vi "HFRR ADV v015 new software.vi"() -> ()   [LabVIEW 2025] (continued)
              n2034 = String Subset(string=w2234, offset (0)=35, length (rest)=9 ("length (rest)")) -> (substring=w2257:string)
              n2035 = String Subset(string=w2234, offset (0)=55, length (rest)=9 ("length (rest)")) -> (substring=w2242:string)
              n2036 = String Subset(string=w2234, offset (0)=25) -> (substring=w2238:string)  [unwired: 1 in]
              n2037 = String Subset(string=w2234, offset (0)=15, length (rest)=9 ("length (rest)")) -> (substring=w2263:string)
              n2038 = String Subset(string=w2234, offset (0)=0, length (rest)=14 ("length (rest)")) -> (substring=w2260:string)
              n2039 = String Subset(string=w2234, offset (0)=45, length (rest)=9 ("length (rest)")) -> (substring=w2247:string)
              n2040 = String Subset(string=w2234, offset (0)=65, length (rest)=9 ("length (rest)")) -> (substring=w2253:string)
              n2041 = Fract/Exp String To Number(string=w2236) -> (number=w2233:dbl)  [unwired: 3 in, 1 out]
              n2042 = Fract/Exp String To Number(string=w2257) -> (number=w2255:dbl)  [unwired: 3 in, 1 out]
              n2043 = Fract/Exp String To Number(string=w2242) -> (number=w2240:dbl)  [unwired: 3 in, 1 out]
              n2044 = Fract/Exp String To Number(string=w2238) -> (number=w2237:dbl)  [unwired: 3 in, 1 out]
              n2045 = Fract/Exp String To Number(string=w2263) -> (number=w2254:dbl)  [unwired: 3 in, 1 out]
              n2046 = Fract/Exp String To Number(string=w2260) -> (number=w2256:dbl)  [unwired: 3 in, 1 out]
              n2047 = Fract/Exp String To Number(string=w2247) -> (number=w2244:dbl)  [unwired: 3 in, 1 out]
              n2048 = Fract/Exp String To Number(string=w2253) -> (number=w2250:dbl)  [unwired: 3 in, 1 out]
              n2049 = Add(x=w2250, y=0.0) -> (x+y=w2248:dbl)
            }
            n2050 = String To Path(string=w2093) -> (path=w2191:path)
            n2051 = String To Path(string=w2091) -> (path=w2185:path)
            n2052 = local read "Numeric 11"() -> (w2175:i32)
            n2053 = local read "Numeric 13"() -> (w2177:i32)
            n2054 = Open/Create/Replace File "Open File"(file path (use dialog)=w2191) -> (refnum out=w2189:refnum<file>, error out=w2188:errorcluster)  [unwired: 5 in, 1 out]
            n2055 = Open/Create/Replace File "Open File"(file path (use dialog)=w2185) -> (refnum out=w2184:refnum<file>, error out=w2183:errorcluster)  [unwired: 5 in, 1 out]
            n2056 = for {
              N: w2175 -> [_]
              tunnel: w2189 -> [w2304]
              tunnel: w2188 -> [w2303]
              tunnel: [w2293] -> w2155 mode=indexing
              tunnel: [w2291] -> w2153 mode=indexing
              tunnel: [w2292] -> w2148 mode=indexing
              tunnel: w2174 -> [_]
              tunnel: [w2285] -> w2150 mode=indexing
              tunnel: [w2281] -> w2126 mode=indexing
              tunnel: [w2277] -> w2101 mode=indexing
              tunnel: [w2273] -> w2082 mode=indexing
              tunnel: [w2268] -> w2040 mode=indexing
              (unwired) TRUE ("line mode (F)")
              n2057 = Read from Text File "Read File"(file (use dialog)=w2304, error in=w2303) -> (text=w2269:string)  [unwired: 2 in, 3 out]
              n2058 = local write "String 7"(w2269) -> ()
              n2059 = String Subset(string=w2269, offset (0)=85, length (rest)=9 ("length (rest)")) -> (substring=w2272:string)
              n2060 = String Subset(string=w2269, offset (0)=35, length (rest)=9 ("length (rest)")) -> (substring=w2294:string)
              n2061 = String Subset(string=w2269, offset (0)=55, length (rest)=9 ("length (rest)")) -> (substring=w2280:string)
              n2062 = String Subset(string=w2269, offset (0)=25, length (rest)=9 ("length (rest)")) -> (substring=w2274:string)
              n2063 = String Subset(string=w2269, offset (0)=45, length (rest)=9 ("length (rest)")) -> (substring=w2282:string)
              n2064 = String Subset(string=w2269, offset (0)=0, length (rest)=14 ("length (rest)")) -> (substring=w2297:string)
              n2065 = String Subset(string=w2269, offset (0)=15, length (rest)=9 ("length (rest)")) -> (substring=w2300:string)
              n2066 = String Subset(string=w2269, offset (0)=65, length (rest)=9 ("length (rest)")) -> (substring=w2286:string)
              n2067 = Fract/Exp String To Number(string=w2272) -> (number=w2268:dbl)  [unwired: 3 in, 1 out]
              n2068 = Fract/Exp String To Number(string=w2294) -> (number=w2292:dbl)  [unwired: 3 in, 1 out]
              n2069 = Fract/Exp String To Number(string=w2280) -> (number=w2277:dbl)  [unwired: 3 in, 1 out]
              n2070 = Fract/Exp String To Number(string=w2274) -> (number=w2273:dbl)  [unwired: 3 in, 1 out]
              n2071 = Fract/Exp String To Number(string=w2282) -> (number=w2281:dbl)  [unwired: 3 in, 1 out]
              n2072 = Fract/Exp String To Number(string=w2297) -> (number=w2293:dbl)  [unwired: 3 in, 1 out]
              n2073 = Fract/Exp String To Number(string=w2300) -> (number=w2291:dbl)  [unwired: 3 in, 1 out]
              n2074 = Fract/Exp String To Number(string=w2286) -> (number=w2289:dbl)  [unwired: 3 in, 1 out]
              n2075 = Add(x=w2289, y=0.0) -> (x+y=w2285:dbl)
            }
            n2076 = for {
              N: w2177 -> [_]
              tunnel: w2184 -> [w2232]
              tunnel: w2183 -> [w2231]
              tunnel: [w2221] -> w2137 mode=indexing
              tunnel: [w2220] -> w2130 mode=indexing
              tunnel: w2174 -> [_]
              tunnel: [w2209] -> w2135 mode=indexing
              tunnel: [w2214] -> w2132 mode=indexing
              tunnel: [w2210] -> w2122 mode=indexing
              tunnel: [w2205] -> w2097 mode=indexing
              tunnel: [w2201] -> w2078 mode=indexing
              tunnel: [w2196] -> w2038 mode=indexing
              (unwired) 1.0 ("x")
              (unwired) TRUE ("line mode (F)")
              n2077 = Read from Text File "Read File"(file (use dialog)=w2232, error in=w2231) -> (text=w2197:string)  [unwired: 2 in, 3 out]
              n2078 = local write "String 12"(w2197) -> ()
              n2079 = String Subset(string=w2197, offset (0)=85, length (rest)=9 ("length (rest)")) -> (substring=w2199:string)
              n2080 = String Subset(string=w2197, offset (0)=35, length (rest)=9 ("length (rest)")) -> (substring=w2222:string)
              n2081 = String Subset(string=w2197, offset (0)=55, length (rest)=9 ("length (rest)")) -> (substring=w2207:string)
              n2082 = String Subset(string=w2197, offset (0)=25, length (rest)=9 ("length (rest)")) -> (substring=w2203:string)
              n2083 = String Subset(string=w2197, offset (0)=45, length (rest)=9 ("length (rest)")) -> (substring=w2212:string)
              n2084 = String Subset(string=w2197, offset (0)=15, length (rest)=9 ("length (rest)")) -> (substring=w2228:string)
              n2085 = String Subset(string=w2197, offset (0)=0, length (rest)=14 ("length (rest)")) -> (substring=w2225:string)
              n2086 = String Subset(string=w2197, offset (0)=65, length (rest)=9 ("length (rest)")) -> (substring=w2215:string)
              n2087 = Fract/Exp String To Number(string=w2199) -> (number=w2196:dbl)  [unwired: 3 in, 1 out]
              n2088 = Fract/Exp String To Number(string=w2222) -> (number=w2220:dbl)  [unwired: 3 in, 1 out]
              n2089 = Fract/Exp String To Number(string=w2207) -> (number=w2205:dbl)  [unwired: 3 in, 1 out]
              n2090 = Fract/Exp String To Number(string=w2203) -> (number=w2201:dbl)  [unwired: 3 in, 1 out]
              n2091 = Fract/Exp String To Number(string=w2212) -> (number=w2210:dbl)  [unwired: 3 in, 1 out]
              n2092 = Fract/Exp String To Number(string=w2228) -> (number=w2209:dbl)  [unwired: 3 in, 1 out]
              n2093 = Fract/Exp String To Number(string=w2225) -> (number=w2221:dbl)  [unwired: 3 in, 1 out]
              n2094 = Fract/Exp String To Number(string=w2215) -> (number=w2218:dbl)  [unwired: 3 in, 1 out]
              n2095 = Add(x=w2218, y=0.0) -> (x+y=w2214:dbl)
            }
            n2096 = Delete From Array(array=w2080, index=0) -> (array with subset deleted=w2053:dbl[])  [unwired: 1 in, 1 out]
            n2097 = Delete From Array(array=w2143, index=0) -> (array with subset deleted=w2116:dbl[])  [unwired: 1 in, 1 out]
            n2098 = Delete From Array(array=w2123, index=0) -> (array with subset deleted=w2111:dbl[])  [unwired: 1 in, 1 out]
            n2099 = Delete From Array(array=w2141, index=0) -> (array with subset deleted=w2142:dbl[])  [unwired: 1 in, 1 out]
            n2100 = call-poly <vilib>:"Mean.vi"("X"=w2053) -> ("mean"=→"КОФ2 4":dbl)  [unwired: 1 out]
            n2101 = call-poly <vilib>:"Mean.vi"("X"=w2116) -> ("mean"=→"КОФ3":dbl)  [unwired: 1 out]
            n2102 = call-poly <vilib>:"Mean.vi"("X"=w2111) -> ("mean"=→"CP3":dbl)  [unwired: 1 out]
            n2103 = Delete From Array(array=w2105, index=0) -> (array with subset deleted=w2032:dbl[])  [unwired: 1 in, 1 out]
            n2104 = Delete From Array(array=w2044, index=0) -> (array with subset deleted=w2031:dbl[])  [unwired: 1 in, 1 out]
            n2105 = Delete From Array(array=w2084, index=0) -> (array with subset deleted=w2055:dbl[])  [unwired: 1 in, 1 out]
            n2106 = Delete From Array(array=w2162, index=0) -> (array with subset deleted=w2117:dbl[])  [unwired: 1 in, 1 out]
            n2107 = Delete From Array(array=w2128, index=0) -> (array with subset deleted=w2113:dbl[])  [unwired: 1 in, 1 out]
            "array w/ subset deleted" <- w2113
            n2108 = Delete From Array(array=w2159, index=0) -> (array with subset deleted=w2160:dbl[])  [unwired: 1 in, 1 out]
            n2109 = call-poly <vilib>:"Mean.vi"("X"=w2055) -> ("mean"=→"КОФ2 2":dbl)  [unwired: 1 out]
            n2110 = call-poly <vilib>:"Mean.vi"("X"=w2117) -> ("mean"=→"КОФ1":dbl)  [unwired: 1 out]
            n2111 = Bundle "Bundle"(w2032, w2031) -> (w2037:cluster{dbl[], dbl[]})  [unwired: 1 in]
            n2112 = Bundle "Bundle"(w2032, w2160) -> (w2024:cluster{dbl[], dbl[]})  [unwired: 1 in]
            n2113 = Delete From Array(array=w2039, index=0) -> (array with subset deleted=w2027:dbl[])  [unwired: 1 in, 1 out]
            n2114 = Delete From Array(array=w2040, index=0) -> (array with subset deleted=w2029:dbl[])  [unwired: 1 in, 1 out]
            n2115 = Delete From Array(array=w2150, index=0) -> (array with subset deleted=w2151:dbl[])  [unwired: 1 in, 1 out]
            n2116 = Delete From Array(array=w2038, index=0) -> (array with subset deleted=w2025:dbl[])  [unwired: 1 in, 1 out]
            n2117 = Delete From Array(array=w2132, index=0) -> (array with subset deleted=w2133:dbl[])  [unwired: 1 in, 1 out]
            n2118 = Delete From Array(array=w2157, index=0) -> (array with subset deleted=w2063:dbl[])  [unwired: 1 in, 1 out]
            n2119 = Delete From Array(array=w2103, index=0) -> (array with subset deleted=w2059:dbl[])  [unwired: 1 in, 1 out]
            n2120 = Delete From Array(array=w2139, index=0) -> (array with subset deleted=w2061:dbl[])  [unwired: 1 in, 1 out]
            n2121 = Delete From Array(array=w2099, index=0) -> (array with subset deleted=w2057:dbl[])  [unwired: 1 in, 1 out]
            n2122 = Delete From Array(array=w2148, index=0) -> (array with subset deleted=w2062:dbl[])  [unwired: 1 in, 1 out]
            n2123 = Delete From Array(array=w2101, index=0) -> (array with subset deleted=w2058:dbl[])  [unwired: 1 in, 1 out]
            n2124 = Delete From Array(array=w2082, index=0) -> (array with subset deleted=w2054:dbl[])  [unwired: 1 in, 1 out]
            n2125 = Delete From Array(array=w2126, index=0) -> (array with subset deleted=w2112:dbl[])  [unwired: 1 in, 1 out]
            n2126 = Delete From Array(array=w2153, index=0) -> (array with subset deleted=w2114:dbl[])  [unwired: 1 in, 1 out]
            n2127 = Delete From Array(array=w2130, index=0) -> (array with subset deleted=w2060:dbl[])  [unwired: 1 in, 1 out]
            n2128 = Delete From Array(array=w2097, index=0) -> (array with subset deleted=w2056:dbl[])  [unwired: 1 in, 1 out]
            n2129 = Delete From Array(array=w2078, index=0) -> (array with subset deleted=w2052:dbl[])  [unwired: 1 in, 1 out]
            n2130 = Delete From Array(array=w2122, index=0) -> (array with subset deleted=w2110:dbl[])  [unwired: 1 in, 1 out]
            n2131 = Delete From Array(array=w2135, index=0) -> (array with subset deleted=w2115:dbl[])  [unwired: 1 in, 1 out]
            n2132 = Delete From Array(array=w2145, index=0) -> (array with subset deleted=w2028:dbl[])  [unwired: 1 in, 1 out]
            n2133 = Delete From Array(array=w2155, index=0) -> (array with subset deleted=w2030:dbl[])  [unwired: 1 in, 1 out]
            n2134 = Delete From Array(array=w2137, index=0) -> (array with subset deleted=w2026:dbl[])  [unwired: 1 in, 1 out]
            n2135 = Bundle "Bundle"(w2032, w2063) -> (w2050:cluster{dbl[], dbl[]})  [unwired: 1 in]
            n2136 = Bundle "Bundle"(w2032, w2117) -> (w2051:cluster{dbl[], dbl[]})  [unwired: 1 in]
            n2137 = Bundle "Bundle"(w2063, w2059) -> (w2065:cluster{dbl[], dbl[]})  [unwired: 1 in]
            n2138 = Bundle "Bundle"(w2028, w2027) -> (w2035:cluster{dbl[], dbl[]})  [unwired: 1 in]
            n2139 = Bundle "Bundle"(w2061, w2057) -> (w2067:cluster{dbl[], dbl[]})  [unwired: 1 in]
            n2140 = Bundle "Bundle"(w2028, w2061) -> (w2171:cluster{dbl[], dbl[]})  [unwired: 1 in]
            n2141 = Bundle "Bundle"(w2028, w2057) -> (w2095:cluster{dbl[], dbl[]})  [unwired: 1 in]
            n2142 = Bundle "Bundle"(w2028, w2116) -> (w2181:cluster{dbl[], dbl[]})  [unwired: 1 in]
            n2143 = Bundle "Bundle"(w2028, w2111) -> (w2119:cluster{dbl[], dbl[]})  [unwired: 1 in]
            n2144 = Bundle "Bundle"(w2028, w2142) -> (w2166:cluster{dbl[], dbl[]})  [unwired: 1 in]
            n2145 = Bundle "Bundle"(w2062, w2058) -> (w2066:cluster{dbl[], dbl[]})  [unwired: 1 in]
            n2146 = Bundle "Bundle"(w2030, w2029) -> (w2036:cluster{dbl[], dbl[]})  [unwired: 1 in]
            n2147 = Bundle "Bundle"(w2030, w2062) -> (w2173:cluster{dbl[], dbl[]})  [unwired: 1 in]
            n2148 = Bundle "Bundle"(w2030, w2058) -> (w2096:cluster{dbl[], dbl[]})  [unwired: 1 in]
            n2149 = Bundle "Bundle"(w2030, w2112) -> (w2120:cluster{dbl[], dbl[]})  [unwired: 1 in]
            n2150 = Bundle "Bundle"(w2030, w2114) -> (w2182:cluster{dbl[], dbl[]})  [unwired: 1 in]
            n2151 = Bundle "Bundle"(w2030, w2151) -> (w2164:cluster{dbl[], dbl[]})  [unwired: 1 in]
            n2152 = Bundle "Bundle"(w2060, w2056) -> (w2068:cluster{dbl[], dbl[]})  [unwired: 1 in]
            n2153 = Bundle "Bundle"(w2026, w2025) -> (w2034:cluster{dbl[], dbl[]})  [unwired: 1 in]
            n2154 = Bundle "Bundle"(w2026, w2060) -> (w2172:cluster{dbl[], dbl[]})  [unwired: 1 in]
            n2155 = Bundle "Bundle"(w2026, w2056) -> (w2094:cluster{dbl[], dbl[]})  [unwired: 1 in]
            n2156 = Bundle "Bundle"(w2026, w2110) -> (w2118:cluster{dbl[], dbl[]})  [unwired: 1 in]
            n2157 = Bundle "Bundle"(w2026, w2115) -> (w2180:cluster{dbl[], dbl[]})  [unwired: 1 in]
            n2158 = Bundle "Bundle"(w2026, w2133) -> (w2165:cluster{dbl[], dbl[]})  [unwired: 1 in]
            n2159 = call-poly <vilib>:"Mean.vi"("X"=w2113) -> ("mean"=→"CP1":dbl)  [unwired: 1 out]
            n2160 = call-poly <vilib>:"Mean.vi"("X"=w2054) -> ("mean"=→"КОФ2 3":dbl)  [unwired: 1 out]
            n2161 = call-poly <vilib>:"Mean.vi"("X"=w2112) -> ("mean"=→"CP2":dbl)  [unwired: 1 out]
            n2162 = call-poly <vilib>:"Mean.vi"("X"=w2114) -> ("mean"=→"КОФ2":dbl)  [unwired: 1 out]
            n2163 = call-poly <vilib>:"Mean.vi"("X"=w2052) -> ("mean"=→"КОФ2 5":dbl)  [unwired: 1 out]
            n2164 = call-poly <vilib>:"Mean.vi"("X"=w2110) -> ("mean"=→"CP4":dbl)  [unwired: 1 out]
            n2165 = call-poly <vilib>:"Mean.vi"("X"=w2115) -> ("mean"=→"КОФ4":dbl)  [unwired: 1 out]
            n2166 = Bundle "Bundle"(w2032, w2059) -> (w2023:cluster{dbl[], dbl[]})  [unwired: 1 in]
            n2167 = Bundle "Bundle"(w2032, w2113) -> (w2046:cluster{dbl[], dbl[]})  [unwired: 1 in]
            n2168 = Build Array "Build Array"(w2023, w2046) -> (w2049:cluster{dbl[], dbl[]}[])
            "XY Graph 17" <- w2049
            n2169 = Build Array "Build Array"(w2037, w2036, w2035, w2034) -> (→"Frequency ( Hz )":cluster{dbl[], dbl[]}[])
            n2170 = Build Array "Build Array"(w2065, w2066, w2067, w2068) -> (→"Air Temp ( °C ) vs Humidity ( % RH )":cluster{dbl[], dbl[]}[])
            n2171 = Build Array "Build Array"(w2050, w2173, w2171, w2172) -> (→"Air Temperature  ( °C )":cluster{dbl[], dbl[]}[])
            n2172 = Build Array "Build Array"(w2023, w2096, w2095, w2094) -> (→"Humidity ( %RH )":cluster{dbl[], dbl[]}[])
            n2173 = Build Array "Build Array"(w2051, w2182, w2181, w2180) -> (→"Coefficient Of Friction":cluster{dbl[], dbl[]}[])
            n2174 = Build Array "Build Array"(w2046, w2120, w2119, w2118) -> (→"Sample Temperature ( °C )":cluster{dbl[], dbl[]}[])
            n2175 = Build Array "Build Array"(w2024, w2164, w2166, w2165) -> (→"XY Graph 13":cluster{dbl[], dbl[]}[])
            n2176 = Bundle "Bundle"(w2032, w2055) -> (w2077:cluster{dbl[], dbl[]})  [unwired: 1 in]
            n2177 = Bundle "Bundle"(w2028, w2053) -> (w2075:cluster{dbl[], dbl[]})  [unwired: 1 in]
            n2178 = Bundle "Bundle"(w2030, w2054) -> (w2076:cluster{dbl[], dbl[]})  [unwired: 1 in]
            n2179 = Bundle "Bundle"(w2026, w2052) -> (w2074:cluster{dbl[], dbl[]})  [unwired: 1 in]
            n2180 = Build Array "Build Array"(w2077, w2076, w2075, w2074) -> (→"Stroke ( mm )":cluster{dbl[], dbl[]}[])
            n2181 = local write "XY Graph 16"(w2049) -> ()
          }
          frame #2 {
          }
          frame #3 {
            n2182 = local write "Numeric 8"(0 ("Numeric 8")) -> ()
            n2183 = local write "Numeric 11"(0 ("Numeric 11")) -> ()
            n2184 = local write "Numeric 12"(0 ("Numeric 12")) -> ()
            n2185 = local write "Numeric 13"(0 ("Numeric 13")) -> ()
            n2186 = property on="OPEN" class="Bool (strict)"("Visible"=TRUE) -> ()  [unwired: 2 in, 2 out]
            n2187 = local read "String Control 2"() -> (w2349:string)
            n2188 = local read "String Control 4"() -> (w2348:string)
            n2189 = local read "String Control 6"() -> (w2347:string)
            n2190 = local read "String Control 8"() -> (w2346:string)
            n2191 = Match Pattern(string=w2349, regular expression="Samples / cycle :- ") -> (after substring=w2363:string)  [unwired: 1 in, 3 out]
            n2192 = Match Pattern(string=w2349, regular expression="Frequency :- ") -> (after substring=w2382:string)  [unwired: 1 in, 3 out]
            n2193 = Match Pattern(string=w2348, regular expression="Samples / cycle :- ") -> (after substring=w2359:string)  [unwired: 1 in, 3 out]
            n2194 = Match Pattern(string=w2348, regular expression="Frequency :- ") -> (after substring=w2377:string)  [unwired: 1 in, 3 out]
            n2195 = Match Pattern(string=w2347, regular expression="Samples / cycle :- ") -> (after substring=w2355:string)  [unwired: 1 in, 3 out]
            n2196 = Match Pattern(string=w2347, regular expression="Frequency :- ") -> (after substring=w2372:string)  [unwired: 1 in, 3 out]
            n2197 = Match Pattern(string=w2346, regular expression="Samples / cycle :- ") -> (after substring=w2351:string)  [unwired: 1 in, 3 out]
            n2198 = Match Pattern(string=w2346, regular expression="Frequency :- ") -> (after substring=w2367:string)  [unwired: 1 in, 3 out]
            n2199 = String Subset(string=w2363, length (rest)=6 ("length (rest)")) -> (substring=w2365:string)  [unwired: 1 in]
            n2200 = String Subset(string=w2382, length (rest)=9 ("length (rest)")) -> (substring=w2384:string)  [unwired: 1 in]
            n2201 = String Subset(string=w2359, length (rest)=6 ("length (rest)")) -> (substring=w2361:string)  [unwired: 1 in]
            n2202 = String Subset(string=w2377, length (rest)=9 ("length (rest)")) -> (substring=w2379:string)  [unwired: 1 in]
            n2203 = String Subset(string=w2355, length (rest)=6 ("length (rest)")) -> (substring=w2357:string)  [unwired: 1 in]
            n2204 = String Subset(string=w2372, length (rest)=9 ("length (rest)")) -> (substring=w2374:string)  [unwired: 1 in]
            n2205 = String Subset(string=w2351, length (rest)=6 ("length (rest)")) -> (substring=w2353:string)  [unwired: 1 in]
            n2206 = String Subset(string=w2367, length (rest)=9 ("length (rest)")) -> (substring=w2369:string)  [unwired: 1 in]
            n2207 = Fract/Exp String To Number(string=w2365) -> (number=w2345:dbl)  [unwired: 3 in, 1 out]
            n2208 = Fract/Exp String To Number(string=w2384) -> (number=w2385:dbl)  [unwired: 3 in, 1 out]
            n2209 = Fract/Exp String To Number(string=w2361) -> (number=w2344:dbl)  [unwired: 3 in, 1 out]
            n2210 = Fract/Exp String To Number(string=w2379) -> (number=w2380:dbl)  [unwired: 3 in, 1 out]
            n2211 = Fract/Exp String To Number(string=w2357) -> (number=w2343:dbl)  [unwired: 3 in, 1 out]
            n2212 = Fract/Exp String To Number(string=w2374) -> (number=w2375:dbl)  [unwired: 3 in, 1 out]
            n2213 = Fract/Exp String To Number(string=w2353) -> (number=w2342:dbl)  [unwired: 3 in, 1 out]
            n2214 = Fract/Exp String To Number(string=w2369) -> (number=w2370:dbl)  [unwired: 3 in, 1 out]
            n2215 = local write "sample1"(w2345) -> ()
            n2216 = local write "freq1"(w2385) -> ()
            n2217 = local write "sample2"(w2344) -> ()
            n2218 = local write "freq2"(w2380) -> ()
            n2219 = local write "sample3"(w2343) -> ()
            n2220 = local write "freq3"(w2375) -> ()
            n2221 = local write "sample4"(w2342) -> ()
            n2222 = local write "freq 4"(w2370) -> ()
          }
        }
      }
    }
    n2223 = case shown="True" w1834 {
      selector: w1834 -> [_ w1962]
      frame False {
      }
      frame True {
        n2224 = Not(x=w1962) -> (.not. x?=w1958:bool)
        n2225 = local write "service 3"(w1958) -> ()
        n2226 = local write "OPEN 6"(w1958) -> ()
        n2227 = call <vilib>:"System Exec.vi"("wait until completion? (T)"=TRUE, "command line"="C:\\LAB-IQ\\Scar View.exe") -> ("error out"=→"error out 5":errorcluster)  [unwired: 6 in, 3 out]
      }
    }
    n2228 = case shown="\"Acquire\", Default" w1845 {
      frame "Acquire", Default {
        w2858 = 0.2 ("y")
        w2863 = 1.0 ("y")
        w2864 = 0.8 ("y")
        # "Elapsed time\ncof\nstroke\nAir temp\nTemp\nHumidity"
        n2229 = disable-structure shown="Disabled" {
          frame Disabled {
            n2230 = local read "Flag"() -> (w2881:dbl)
            n2231 = local read "RUN"() -> (w2878:bool)
            n2232 = Not(x=w2878) -> (.not. x?=w2877:bool)
            n2233 = Equal?(x=w2881, y=10.0) -> (x = y?=w2879:bool)
            n2234 = And(x=w2879, y=w2877) -> (x .and. y?=w2876:bool)
            n2235 = case shown="True" w2876 {
              frame False {
              }
              frame True {
                w2882 = FALSE ("Heater Button")
                n2236 = local write "Humidity"(w2882) -> ()
                n2237 = local write "Heater Button"(w2882) -> ()
              }
            }
          }
          frame Enabled {
          }
        }
        n2238 = disable-structure shown="Disabled" {
          frame Disabled {
            n2239 = case shown="True" {
              selector: _ -> [_ _]
              frame False {
              }
              frame True {
                w2973 = TRUE ("Heater")
                n2240 = local write "Humidity"(w2973) -> ()
                n2241 = local write "Heater Button"(w2973) -> ()
                n2242 = local read "TEST STANDARD"() -> (w2976:T3)
                n2243 = local read "TEST STANDARD"() -> (w2971:T3)
                n2244 = Equal?(x=w2976, y=enum16{"ASTM D6079", "ISO 12156", "Custom"}."ISO 12156" ("Test Standard")) -> (x = y?=w2974:bool)
                n2245 = Equal?(x=w2971, y=enum16{"ASTM D6079", "ISO 12156", "Custom"}."ASTM D6079" ("Test Standard")) -> (x = y?=w2970:bool)
                n2246 = case shown="True" w2974 {
                  frame False {
                  }
                  frame True {
                    n2247 = local write "Heater"(TRUE ("Heater")) -> ()
                    n2248 = local write "airtempflg"(FALSE ("airtempflg")) -> ()
                  }
                }
                n2249 = case shown="True" w2970 {
                  frame False {
                  }
                  frame True {
                    n2250 = local write "Heater"(FALSE ("Heater")) -> ()
                    n2251 = local write "airtempflg"(TRUE ("airtempflg")) -> ()
                  }
                }
              }
            }
          }
          frame Enabled {
          }
        }
        n2252 = stacked-sequence {
          frame #0 {
            n2253 = case shown="True" "RST FF" {
              frame False {
              }
              frame True {
                w3039 = 0.0 ("X Scale.Range:Maximum")
                n2254 = property on="Frictional Force ( N )" class="WFChart (strict)"("XScale.Maximum"=600.0 ("X Scale.Range:Maximum"), "XScale.Minimum"=w3039, "YScale.Maximum"=10.0 ("Y Scale.Range:Maximum"), "YScale.Minimum"=w3039) -> ()  [unwired: 2 in, 2 out]
              }
            }
          }
          frame #1 {
            n2255 = case shown="True" "RST TEMP" {
              frame False {
              }
              frame True {
                n2256 = property on="Temperature ( Deg C )" class="WFChart (strict)"("XScale.Minimum"=0.0 ("X Scale.Range:Minimum"), "XScale.Maximum"=600.0 ("X Scale.Range:Maximum"), "YScale.Minimum"=0.0 ("Y Scale.Range:Minimum"), "YScale.Maximum"=100.0 ("Y Scale.Range:Maximum")) -> ()  [unwired: 2 in, 2 out]
              }
            }
          }
          frame #2 {
            n2257 = case shown="True" "RSTCOF" {
              frame False {
              }
              frame True {
                n2258 = property on="Coefficient of Friction" class="WFChart (strict)"("XScale.Minimum"=0.0 ("X Scale.Range:Minimum"), "XScale.Maximum"=600.0 ("X Scale.Range:Maximum"), "YScale.Maximum"=1.0 ("X Scale.Range:Minimum"), "YScale.Minimum"=0.0 ("X Scale.Range:Minimum")) -> ()  [unwired: 2 in, 2 out]
              }
            }
          }
          frame #3 {
            n2259 = case shown="True" "RSTCOF 2" {
              frame False {
              }
              frame True {
                (unwired) 100.0 ("Y Scale.Range:Maximum")
                (unwired) 0.0 ("Y Scale.Range:Minimum")
                (unwired) 600.0 ("X Scale.Range:Maximum")
                (unwired) 0.0 ("X Scale.Range:Minimum")
              }
            }
          }
          frame #4 {
            n2260 = case shown="True" "RSTCOF 3" {
              frame False {
              }
              frame True {
                n2261 = property on="Electrical Contact Resistance ( % )" class="WFChart (strict)"("XScale.Minimum"=0.0 ("X Scale.Range:Minimum"), "XScale.Maximum"=600.0 ("X Scale.Range:Maximum"), "YScale.Minimum"=0.0 ("Y Scale.Range:Minimum"), "YScale.Maximum"=100.0 ("Y Scale.Range:Maximum")) -> ()  [unwired: 2 in, 2 out]
              }
            }
          }
        }
        n2262 = disable-structure shown="Disabled" {
          frame Disabled {
            n2263 = case shown="True" {
              selector: _ -> [_ _]
              frame False {
              }
              frame True {
                n2264 = local read "zflag 2"() -> (w2940:dbl)
                n2265 = local read "yflag"() -> (w2942:dbl)
                n2266 = Equal?(x=w2942, y=2.0 ("tflag")) -> (x = y?=w2944:bool)
                n2267 = Equal?(x=w2940, y=3.0 ("tflag")) -> (x = y?=w2943:bool)
                n2268 = And(x=w2944, y=w2943) -> (x .and. y?=w2938:bool)
                n2269 = case shown="True" w2938 {
                  frame False {
                  }
                  frame True {
                    w2969 = 0.0 ("zflag")
                    n2270 = local write "zflag"(w2969) -> ()
                    n2271 = local write "zflag 2"(w2969) -> ()
                    n2272 = Delete(path (use dialog)=path "C:/LAB-IQ-NXT/WO 2449 TT.sig" ("file path (dialog if empty)")) -> (deleted path=w2968:path)  [unwired: 4 in, 2 out]
                    n2273 = Delete(path (use dialog)=path "C:/LAB-IQ-NXT/WO 2449 TRH.sig" ("file path (dialog if empty)")) -> (deleted path=w2963:path)  [unwired: 4 in, 2 out]
                    n2274 = local read "SEN.RUN HRS"() -> (w2955:dbl)
                    n2275 = local read "SENSOR TIME"() -> (w2953:dbl)
                    n2276 = call <vilib>:"compatOverwrite.vi"("overwrite (F)"=TRUE) -> ("overwrite?"=w2945:T30)
                    n2277 = call <vilib>:"compatOverwrite.vi"("overwrite (F)"=TRUE) -> ("overwrite?"=w2949:T30)
                    n2278 = local read "Total No. of Tests"() -> (w2956:dbl)
                    n2279 = Add(x=w2953, y=w2955) -> (x+y=w2954:dbl)
                    "SEN.RUN HRS" <- w2954
                    n2280 = Open/Create/Replace File(file path (use dialog)=w2968, operation (0:open)=w2945) -> (refnum out=w2946:refnum<file>, error out=w2947:errorcluster)  [unwired: 4 in, 1 out]
                    n2281 = Open/Create/Replace File(file path (use dialog)=w2963, operation (0:open)=w2949) -> (refnum out=w2950:refnum<file>, error out=w2951:errorcluster)  [unwired: 4 in, 1 out]
                    n2282 = Deny Access(4:w2947, 6:T28."deny none" ("deny mode (2)"), 7:w2946) -> (3:w2967:refnum<file>)  [unwired: 1 out]
                    n2283 = Deny Access(4:w2951, 6:T28."deny none" ("deny mode (2)"), 7:w2950) -> (3:w2959:refnum<file>)  [unwired: 1 out]
                    n2284 = Number To Decimal String(number=w2956) -> (decimal integer string=w2964:string)  [unwired: 1 in]
                    n2285 = Number To Decimal String(number=w2954) -> (decimal integer string=w2960:string)  [unwired: 1 in]
                    n2286 = Write to Binary File(file (use dialog)=w2967, data=w2964, 5:FALSE ("prepend array or string size? (T)")) -> ()  [unwired: 3 in, 3 out]
                    n2287 = Write to Binary File(file (use dialog)=w2959, data=w2960, 5:FALSE ("prepend array or string size? (T)")) -> ()  [unwired: 3 in, 3 out]
                  }
                }
              }
            }
          }
          frame Enabled {
          }
        }
        n2288 = local read "RUN"() -> (w2867:bool)
        n2289 = local read "run replace"() -> (w2871:bool)
        n2290 = local read "run replace"() -> (w2870:bool)
        n2291 = case shown="True" w2867 {
          frame False {
            n2292 = local write "run replace"(FALSE ("run replace")) -> ()
          }
          frame True {
            "run replace" <- TRUE ("run replace")
          }
        }
        n2293 = local read "RUN"() -> (w2875:bool)
        n2294 = local read "Set Temp"() -> (w2837:dbl)
        n2295 = local read "SetTemp"() -> (w2839:dbl)
        n2296 = case shown="False" w2875 {
          tunnel: [FALSE ("TEST RUNNING") TRUE ("TEST RUNNING")] -> w2874
          frame False {
            w3058 = 0.0 ("Flag")
            n2297 = local write "Elapsed time"(0.0 ("elapsedtime")) -> ()
            n2298 = local write "Time Remaining"(w3058) -> ()
            n2299 = local write "Flag"(w3058) -> ()
            n2300 = local write "Remaining Time"(w3058) -> ()
          }
          frame True {
            n2301 = local write "Flag"(10.0 ("Flag")) -> ()
          }
        }
        n2302 = case shown="False" w2871 {
          frame False {
            n2303 = local read "zflag"() -> (→"zflag 2":dbl)
            n2304 = local write "yflag"(2.0 ("tflag")) -> ()
            n2305 = local write "FLAG 4"(0.0 ("FLAG")) -> ()
          }
          frame True {
            n2306 = local write "yflag"(1.0 ("tflag")) -> ()
            n2307 = local write "zflag"(3.0 ("zflag")) -> ()
          }
        }
        n2308 = local read "acq 2"() -> (w2869:bool)
        n2309 = local read "AIR TEMP"() -> (w2832:dbl)
        n2310 = local read "Amb temp"() -> (w2836:dbl)
        n2311 = case shown="True" "Save & Continue" {
          frame False {
          }
          frame True {
            "acq 2" <- TRUE ("acq 2")
          }
        }
        n2312 = local read "Set Rh"() -> (w2838:dbl)
        n2313 = Add(x=w2839, y=w2864) -> (x+y=w2865:dbl)
        n2314 = Subtract(x=w2839, y=w2864) -> (x-y=w2866:dbl)
        n2315 = Add(x=w2837, y=w2858) -> (x+y=w2859:dbl)
        n2316 = Subtract(x=w2837, y=w2858) -> (x-y=w2860:dbl)
        n2317 = And(x=w2869, y=w2870) -> (x .and. y?=w2868:bool)
        n2318 = Greater Or Equal?(x=w2832, y=15.0) -> (x >= y?=w2833:bool)
        "powstat" <- w2833
        n2319 = local read "Humidity ( %RH )"() -> (w2835:dbl)
        n2320 = case shown="True" "Save & Continue" {
          frame False {
          }
          frame True {
            n2321 = while {
              tunnel: "0123456789abcdefghijklmnopqrstuvwxyzABCDEFGHIJKLMNOPQRSTUVWXYZ" ("string 2") -> [w3029]
              shift-right: [w3027] -> w3022
              shift-left: "" -> [w3026]
              i -> [w3036]
              stop <- w3035 stop-if-true
              n2322 = Random Number (0-1)() -> (number: 0 to 1=w3030:dbl)
              n2323 = Multiply(x=w3030, y=62.0) -> (x*y=w3032:dbl)
              n2324 = Decrement(x="Length") -> (x-1=w3025:i16)
              n2325 = To Word Integer(number=w3032) -> (16bit integer=w3033:i16)
              n2326 = String Subset(string=w3029, offset (0)=w3033, length (rest)=1 ("length (rest)")) -> (substring=w3028:string)
              n2327 = Greater Or Equal?(x=w3036, y=w3025) -> (x >= y?=w3035:bool)
              n2328 = Concatenate Strings(w3028, w3026) -> (w3027:string)
            }
            n2329 = local write "UUID"(w3022) -> ()
          }
        }
        n2330 = In Range and Coerce(upper limit=w2865, x=w2836, lower limit=w2866) -> (In Range?=w2855:bool)  [unwired: 1 out]
        n2331 = Add(x=w2838, y=w2863) -> (x+y=w2862:dbl)
        n2332 = Subtract(x=w2838, y=w2863) -> (x-y=w2861:dbl)
        n2333 = local read "TEMP"() -> (w2834:dbl)
        n2334 = case shown="True" "Save & Continue" {
          frame False {
          }
          frame True {
            n2335 = local read "Operator ID"() -> (w3353:string)
            n2336 = local read "FILE"() -> (w3359:string)
            n2337 = String Length(string=w3359) -> (length=w3357:i32)
            n2338 = String Length(string=w3353) -> (length=w3354:i32)
            n2339 = Greater?(x=w3357, y=0) -> (0:w3356:bool)
            n2340 = Greater?(x=w3354, y=0) -> (0:w3352:bool)
            n2341 = And(x=w3356, y=w3352) -> (x .and. y?=w3351:bool)
            n2342 = case shown="True" w3351 {
              frame False {
                n2343 = stacked-sequence {
                  frame #0 {
                    n2344 = One Button Dialog(message="Please Enter a File Name and Operator ID to save data !", button name ("OK")="Ok") -> ()  [unwired: 1 out]
                  }
                  frame #1 {
                    n2345 = local write "Save & Continue"(FALSE ("OK Button")) -> ()
                  }
                }
                n2346 = local write "Save & Continue"(FALSE ("OK Button")) -> ()
              }
              frame True {
                n2347 = stacked-sequence {
                  frame #0 {
                    n2348 = local read "FILE"() -> (w3365:string)
                    n2349 = call "file check.vi"("file name in"=w3365) -> ("file name out"=w3364:string)  [unwired: 9 in, 1 out]
                    n2350 = call <vilib>:"Application Directory.vi"() -> ("Application Directory"=w3375:path)
                    n2351 = Build Path(base path=w3375, name or relative path="data") -> (appended path=w3374:path)
                    n2352 = call <vilib>:"Trim Whitespace.vi"("string"=w3364) -> ("trimmed string"=w3372:string)  [unwired: 1 in]
                    n2353 = call <vilib>:"Trim Whitespace.vi"("string"=w3364) -> ("trimmed string"=w3373:string)  [unwired: 1 in]
                    n2354 = List Folder(path=w3374) -> (folder names=w3370:string[])  [unwired: 3 in, 3 out]
                    n2355 = Match Pattern(string=w3372, regular expression="_(") -> (before substring=w3369:string)  [unwired: 1 in, 3 out]
                    n2356 = for {
                      tunnel: w3370 -> [w3384] mode=indexing
                      tunnel: w3369 -> [w3382]
                      shift-right: [w3380] -> w3367
                      shift-left: bool[] [] -> [w3381]
                      n2357 = Match Pattern(string=w3384, regular expression="_(") -> (before substring=w3383:string)  [unwired: 1 in, 3 out]
                      n2358 = Equal?(x=w3383, y=w3382) -> (x = y?=w3379:bool)
                      n2359 = case shown="True" w3379 {
                        tunnel: w3379 -> [_ w3387]
                        tunnel: w3381 -> [w3386 w3389]
                        tunnel: [w3386 w3388] -> w3380
                        frame False {
                        }
                        frame True {
                          n2360 = Insert Into Array(array=w3389, new element=w3387) -> (w3388:bool[])  [unwired: 1 in]
                        }
                      }
                    }
                    n2361 = Equal?(x=w3370, y=w3369) -> (x = y?=w3378:bool[])
                    n2362 = Or Array Elements(Boolean array=w3378) -> (logical OR=w3377:bool)
                    n2363 = Array Size(array=w3367) -> (size(s)=w3366:i32)
                    n2364 = case shown="True" w3377 {
                      tunnel: w3373 -> [_ w3397]
                      tunnel: w3366 -> [_ w3390]
                      frame False {
                      }
                      frame True {
                        n2365 = Number To Decimal String(number=w3390) -> (decimal integer string=w3393:string)  [unwired: 1 in]
                        n2366 = Search/Split String(string=w3397, search string/char (-)="_(" ("regular expression")) -> (substring before match=w3395:string)  [unwired: 1 in, 2 out]
                        n2367 = Concatenate Strings(w3395, "_(" ("regular expression"), w3393, ")" ("regular expression")) -> (w3391:string)
                        n2368 = local write "FILE"(w3391) -> ()
                      }
                    }
                  }
                  frame #1 {
                    w3399 = 0.0
                    w3412 = cluster{"y":dbl, dbl, "y":dbl}[] [] ("History Data")
                    w3413 = FALSE ("Heater Button")
                    (unwired) ")!" ("string")
                    (unwired) ")" ("string")
                    w3411 = dbl[] [] ("History Data")
                    w3417 = "\r"
                    # "C:\\WinDucom\\Data\\"
                    # "C:\\LAB-IQ-NXT\\data"
                    n2369 = local write "Humidity ( %RH )"(w3399) -> ()
                    n2370 = local write "Frequency ( Hz )"(w3399) -> ()
                    n2371 = local write "Stroke 3"(w3399) -> ()
                    n2372 = local write "speedop"(0.0 ("PIDclk 2")) -> ()
                    n2373 = local write "Set Temp 2"(65.0 ("Set Temp 2")) -> ()
                    n2374 = local write "AIR TEMP"(w3399) -> ()
                    n2375 = local write "clk"(0.0 ("clk")) -> ()
                    n2376 = local write "Stroke 4"(w3399) -> ()
                    n2377 = local write "COF 2"(w3399) -> ()
                    n2378 = local write "TEMP"(w3399) -> ()
                    n2379 = local write "ecr 3"(w3399) -> ()
                    n2380 = local write "FF 3"(w3399) -> ()
                    n2381 = local write "FF 2"(w3399) -> ()
                    n2382 = property on="Humidity ( %RH )" class="WFChart (strict)"("History Data"=w3411) -> ()  [unwired: 2 in, 2 out]
                    n2383 = property on="Coefficient of Friction" class="WFChart (strict)"("History Data"=w3411) -> ()  [unwired: 2 in, 2 out]
                    n2384 = property on="Coefficient of Friction" class="WFChart (strict)"("History Data"=w3411) -> ()  [unwired: 2 in, 2 out]
                    n2385 = property on="Frictional Force ( N )" class="WFChart (strict)"("History Data"=w3411) -> ()  [unwired: 2 in, 2 out]
                    n2386 = property on="Electrical Contact Resistance ( % )" class="WFChart (strict)"("History Data"=w3411) -> ()  [unwired: 2 in, 2 out]
                    n2387 = property on="Electrical Contact Resistance ( % )" class="WFChart (strict)"("History Data"=w3411) -> ()  [unwired: 2 in, 2 out]
                    n2388 = property on="Temperature ( Deg C )" class="WFChart (strict)"("History Data"=w3411) -> ()  [unwired: 2 in, 2 out]
                    n2389 = property on="Frictional Force ( N )" class="WFChart (strict)"("History Data"=w3411) -> ()  [unwired: 2 in, 2 out]
                    n2390 = property on="Coefficient of Friction" class="WFChart (strict)"("History Data"=w3411) -> ()  [unwired: 2 in, 2 out]
                    n2391 = property on="Frictional Force ( N )" class="WFChart (strict)"("History Data"=w3411) -> ()  [unwired: 2 in, 2 out]
                    n2392 = property on="Electrical Contact Resistance ( % )" class="WFChart (strict)"("History Data"=w3411) -> ()  [unwired: 2 in, 2 out]
                    n2393 = property on="Temperature ( Deg C )" class="WFChart (strict)"("History Data"=w3411) -> ()  [unwired: 2 in, 2 out]
                    n2394 = property on="Humidity ( %RH )" class="WFChart (strict)"("History Data"=w3411) -> ()  [unwired: 2 in, 2 out]
                    n2395 = property on="Stroke ( mm )" class="WFChart (strict)"("History Data"=w3412) -> ()  [unwired: 2 in, 2 out]
                    n2396 = property on="Stroke ( mm )" class="WFChart (strict)"("History Data"=w3412) -> ()  [unwired: 2 in, 2 out]
                    n2397 = local write "Humidity"(w3413) -> ()
                    n2398 = local write "Heater Button"(w3413) -> ()
                    n2399 = local read "FILE"() -> (w3407:string)
                    n2400 = disable-structure shown="Enabled" {
                      disable-tunnel: [w3452 _] -> w3398
                      frame Enabled {
                        n2401 = local read "NORMAL LOAD"() -> (w3452:dbl)
                      }
                      frame Disabled {
                      }
                    }
                    n2402 = call "file check.vi"("file name in"=w3407) -> ("error out"=w3410:errorcluster, "file name out"=w3404:string)  [unwired: 9 in]
                    n2403 = call "FILE PATH CREATION.vi"("error in"=w3410, "FILE NAME :"=w3404) -> ("FILE OUT"=w3403:path)  [unwired: 8 in, 1 out]
                    n2404 = Concatenate Strings(w3404, ".dgf" ("Substring")) -> (w3409:string)
                    n2405 = Concatenate Strings(w3404, ".duf" ("Substring")) -> (w3405:string)
                    n2406 = Multiply(x=w3398, y=1.0) -> (x*y=w3431:dbl)
                    n2407 = Build Path(base path=w3403, name or relative path=w3409) -> (appended path=w3402:path)
                    n2408 = Build Path(base path=w3403, name or relative path=w3405) -> (appended path=w3401:path)
                    n2409 = Number To Fractional String(number=w3431, width (-)=i16 5, precision (6)=i16 2) -> (F-format string=w3439:string)  [unwired: 1 in]
                    n2410 = local read "Fuel Discription :"() -> (w3427:string)
                    n2411 = local read "Batch Ref Num :"() -> (w3415:string)
                    n2412 = Get Date/Time String(date format (0)=enum16{"short", "long", "abbreviated"}."short") -> (date string=w3450:string, time string=w3447:string)  [unwired: 2 in]
                    n2413 = local read "Remarks :"() -> (w3426:string)
                    n2414 = Concatenate Strings("Load :- " ("Substring"), w3439, " grams ," ("Substring")) -> (w3438:string)
                    n2415 = local read "String 41"() -> (w3418:string)
                    n2416 = Concatenate Strings(w3427) -> (w3428:string)
                    n2417 = Concatenate Strings(w3415) -> (w3414:string)
                    n2418 = Concatenate Strings("tested by") -> (w3422:string)
                    n2419 = Concatenate Strings("(" ("Substring"), w3450, ")" ("Substring"), w3447) -> (w3420:string)
                    "concatenated string" <- w3420
                    n2420 = Concatenate Strings(w3426, "," ("string")) -> (w3425:string)
                    n2421 = Concatenate Strings("  TIME;      COF;       STROKE;     AIR TEMP;  TEMP;  HUMIDITY;  ECR; PID-OUT; FREQUENCY" ("Substring"), "\r") -> (w3434:string)
                    n2422 = Concatenate Strings(w3418, w3417, "Fuel Discription :-" ("Substring"), w3428, w3417, w3438, w3417, "Batch Ref Num :-" ("Substring"), w3414, w3417, " Remarks :- " ("Substring"), w3425, w3417, " Date :- " ("Substring"), w3420, w3417, "Tested By :-" ("Substring"), w3422) -> (w3432:string)
                    "REMARKS" <- w3432
                    n2423 = call <vilib>:"Write Characters To File.vi"("append to file? (new file:F)"=FALSE, "character string"=w3434, "file path (dialog if empty)"=w3402) -> ()  [unwired: 2 in, 1 out]
                    n2424 = call <vilib>:"Write Characters To File.vi"("append to file? (new file:F)"=FALSE, "character string"=w3432, "file path (dialog if empty)"=w3401) -> ()  [unwired: 2 in, 1 out]
                  }
                  frame #2 {
                    n2425 = local write "Cycles elapsed"(0 ("Cycles elapsed")) -> ()
                    n2426 = local write "cyclecount"(0 ("cyclecount")) -> ()
                    n2427 = local write "Save & Continue"(FALSE ("OK")) -> ()
                    n2428 = local write "autostrtflg"(TRUE ("autostrtflg")) -> ()
                    n2429 = local write "Save"(FALSE ("Save")) -> ()
                    n2430 = Get Date/Time In Seconds() -> (seconds since 1Jan1904=w3457:timestamp)
                    n2431 = To Double Precision Float(number=w3457) -> (double precision float=w3456:dbl)
                    n2432 = local write "acq timer"(w3456) -> ()
                    n2433 = One Button Dialog(message="Please ensure sample is mounted properly and machine is ready in all aspects for testing !", button name ("OK")="Ok") -> ()  [unwired: 1 out]
                  }
                  frame #3 {
                    n2434 = stacked-sequence {
                      frame #0 {
                        n2435 = local write "Main Dashboard Buttons"(T1."Dashboard" ("Main Dashboard Buttons")) -> ()
                        n2436 = local write "Main Tab"(T2."Acquire" ("Main Tab")) -> ()
                      }
                      frame #1 {
                        n2437 = local write "EVENT LOG"("" ("EVENT LOG")) -> ()
                      }
                      frame #2 {
                        n2438 = Wait (ms)(milliseconds to wait=u32 50) -> ()  [unwired: 1 out]
                      }
                      frame #3 {
                        n2439 = disable-structure shown="Disabled" {
                          frame Disabled {
                            n2440 = local read "EVENT LOG"() -> (w3469:string)
                            n2441 = call "Event Log.vi"("Content"="Test Details", "EVENT LOG"=w3469) -> ("EVENT LOG"=w3468:string)  [unwired: 8 in, 1 out]
                            n2442 = local write "EVENT LOG"(w3468) -> ()
                          }
                          frame Enabled {
                          }
                        }
                      }
                      frame #4 {
                        n2443 = Wait (ms)(milliseconds to wait=u32 50) -> ()  [unwired: 1 out]
                      }
                      frame #5 {
                        n2444 = local read "FILE"() -> (w3471:string)
                        n2445 = Concatenate Strings("File Name :" ("Content"), w3471) -> (w3472:string)
                        n2446 = local read "EVENT LOG"() -> (w3475:string)
                        n2447 = call "Event Log.vi"("Content"=w3472, "EVENT LOG"=w3475) -> ("EVENT LOG"=w3474:string)  [unwired: 8 in, 1 out]
                        n2448 = local write "EVENT LOG"(w3474) -> ()
                      }
                      frame #6 {
                        n2449 = Wait (ms)(milliseconds to wait=u32 50) -> ()  [unwired: 1 out]
                      }
                      frame #7 {
                        n2450 = local read "Batch Ref Num :"() -> (w3477:string)
                        n2451 = Concatenate Strings("Batch Ref No :" ("Content"), w3477) -> (w3478:string)
                        n2452 = local read "EVENT LOG"() -> (w3481:string)
                        n2453 = call "Event Log.vi"("Content"=w3478, "EVENT LOG"=w3481) -> ("EVENT LOG"=w3480:string)  [unwired: 8 in, 1 out]
                        n2454 = local write "EVENT LOG"(w3480) -> ()
                      }
                      frame #8 {
                        n2455 = Wait (ms)(milliseconds to wait=u32 50) -> ()  [unwired: 1 out]
                      }
                      frame #9 {
                        n2456 = local read "tested by"() -> (w3483:string)
                        n2457 = Concatenate Strings("Tested By :" ("Content"), w3483) -> (w3484:string)
                        n2458 = local read "EVENT LOG"() -> (w3487:string)
                        n2459 = call "Event Log.vi"("Content"=w3484, "EVENT LOG"=w3487) -> ("EVENT LOG"=w3486:string)  [unwired: 8 in, 1 out]
                        n2460 = local write "EVENT LOG"(w3486) -> ()
                      }
                      frame #10 {
                        n2461 = Wait (ms)(milliseconds to wait=u32 50) -> ()  [unwired: 1 out]
                      }
                      frame #11 {
                        n2462 = local read "TEST STANDARD"() -> (w3490:T3)
                        n2463 = case shown="\"ASTM D6079\", Default" w3490 {
                          tunnel: ["ASTM D6079" "ISO 12156" "CEC F-096-A-06" "Custom"] -> w3489
                          frame "ASTM D6079", Default {
                          }
                          frame "ISO 12156" {
                          }
                          frame "CEC F-096-A-06" {
                          }
                          frame "Custom" {
                          }
                        }
                        n2464 = Concatenate Strings("Test Standard :" ("Content"), w3489) -> (w3491:string)
                        n2465 = local read "EVENT LOG"() -> (w3494:string)
                        n2466 = call "Event Log.vi"("Content"=w3491, "EVENT LOG"=w3494) -> ("EVENT LOG"=w3493:string)  [unwired: 8 in, 1 out]
                        n2467 = local write "EVENT LOG"(w3493) -> ()
                      }
                      frame #12 {
                        n2468 = Wait (ms)(milliseconds to wait=u32 50) -> ()  [unwired: 1 out]
                      }
                      frame #13 {
                        n2469 = local read "Fuel Discription :"() -> (w3500:string)
                        n2470 = Concatenate Strings("Fuel Description :" ("Content"), w3500) -> (w3501:string)
                        n2471 = local read "EVENT LOG"() -> (w3504:string)
                        n2472 = call "Event Log.vi"("Content"=w3501, "EVENT LOG"=w3504) -> ("EVENT LOG"=w3503:string)  [unwired: 8 in, 1 out]
                        n2473 = local write "EVENT LOG"(w3503) -> ()
                      }
                      frame #14 {
                        n2474 = Wait (ms)(milliseconds to wait=u32 50) -> ()  [unwired: 1 out]
                      }
                      frame #15 {
                        n2475 = local read "Remarks :"() -> (w3506:string)
                        n2476 = Concatenate Strings("Remarks :" ("Content"), w3506) -> (w3507:string)
                        n2477 = local read "EVENT LOG"() -> (w3510:string)
                        n2478 = call "Event Log.vi"("Content"=w3507, "EVENT LOG"=w3510) -> ("EVENT LOG"=w3509:string)  [unwired: 8 in, 1 out]
                        n2479 = local write "EVENT LOG"(w3509) -> ()
                      }
                      frame #16 {
                        n2480 = Wait (ms)(milliseconds to wait=u32 50) -> ()  [unwired: 1 out]
                      }
                      frame #17 {
                        n2481 = local read "Operator ID"() -> (w3512:string)
                        n2482 = Concatenate Strings("Operator ID :" ("Content"), w3512) -> (w3514:string)
                        n2483 = local read "EVENT LOG"() -> (w3516:string)
                        n2484 = call "Event Log.vi"("Content"=w3514, "EVENT LOG"=w3516) -> ("EVENT LOG"=w3515:string)  [unwired: 8 in, 1 out]
                        n2485 = local write "EVENT LOG"(w3515) -> ()
                      }
                      frame #18 {
                        n2486 = Wait (ms)(milliseconds to wait=u32 50) -> ()  [unwired: 1 out]
                      }
                      frame #19 {
                        n2487 = disable-structure shown="Disabled" {
                          frame Disabled {
                            n2488 = local read "EVENT LOG"() -> (w3520:string)
                            n2489 = call "Event Log.vi"("Content"="Test Parameter", "EVENT LOG"=w3520) -> ("EVENT LOG"=w3519:string)  [unwired: 8 in, 1 out]
                            n2490 = local write "EVENT LOG"(w3519) -> ()
                          }
                          frame Enabled {
                          }
                        }
                      }
                      frame #20 {
                        n2491 = Wait (ms)(milliseconds to wait=u32 50) -> ()  [unwired: 1 out]
                      }
                      frame #21 {
                        n2492 = local read "Set Hz"() -> (w3524:dbl)
                        n2493 = Number To Fractional String(number=w3524, precision (6)=i16 2) -> (F-format string=w3523:string)  [unwired: 2 in]
                        n2494 = Concatenate Strings("Set Frequency [Hz] :" ("Content"), w3523) -> (w3526:string)
                        n2495 = local read "EVENT LOG"() -> (w3528:string)
                        n2496 = call "Event Log.vi"("Content"=w3526, "EVENT LOG"=w3528) -> ("EVENT LOG"=w3527:string)  [unwired: 8 in, 1 out]
                        n2497 = local write "EVENT LOG"(w3527) -> ()
                      }
                      frame #22 {
                        n2498 = Wait (ms)(milliseconds to wait=u32 50) -> ()  [unwired: 1 out]
                      }
                      frame #23 {
                        n2499 = local read "NORMAL LOAD"() -> (w3531:dbl)
                        n2500 = Number To Fractional String(number=w3531, precision (6)=i16 2) -> (F-format string=w3532:string)  [unwired: 2 in]
                        n2501 = Concatenate Strings("Applied Load [grams] :" ("Content"), w3532) -> (w3534:string)
                        n2502 = local read "EVENT LOG"() -> (w3536:string)
                        n2503 = call "Event Log.vi"("Content"=w3534, "EVENT LOG"=w3536) -> ("EVENT LOG"=w3535:string)  [unwired: 8 in, 1 out]
                        n2504 = local write "EVENT LOG"(w3535) -> ()
                      }
                      frame #24 {
                        n2505 = Wait (ms)(milliseconds to wait=u32 50) -> ()  [unwired: 1 out]
                      }
                      frame #25 {
                        n2506 = local read "Set Strk"() -> (w3539:dbl)
                        n2507 = Number To Fractional String(number=w3539, precision (6)=i16 2) -> (F-format string=w3540:string)  [unwired: 2 in]
                        n2508 = Concatenate Strings("Set Stroke [mm] :" ("Content"), w3540) -> (w3542:string)
                        n2509 = local read "EVENT LOG"() -> (w3544:string)
                        n2510 = call "Event Log.vi"("Content"=w3542, "EVENT LOG"=w3544) -> ("EVENT LOG"=w3543:string)  [unwired: 8 in, 1 out]
                        n2511 = local write "EVENT LOG"(w3543) -> ()
                      }
                      frame #26 {
                        n2512 = Wait (ms)(milliseconds to wait=u32 50) -> ()  [unwired: 1 out]
                      }
                      frame #27 {
                        n2513 = local read "Set Temp"() -> (w3547:dbl)
                        n2514 = Number To Fractional String(number=w3547, precision (6)=i16 2) -> (F-format string=w3548:string)  [unwired: 2 in]
                        n2515 = Concatenate Strings("Set Temperature [deg C] :" ("Content"), w3548) -> (w3550:string)
                        n2516 = local read "EVENT LOG"() -> (w3552:string)
                        n2517 = call "Event Log.vi"("Content"=w3550, "EVENT LOG"=w3552) -> ("EVENT LOG"=w3551:string)  [unwired: 8 in, 1 out]
                        n2518 = local write "EVENT LOG"(w3551) -> ()
                      }
                      frame #28 {
                        n2519 = Wait (ms)(milliseconds to wait=u32 50) -> ()  [unwired: 1 out]
                      }
                      frame #29 {
                        n2520 = local read "Set Rh"() -> (w3555:dbl)
                        n2521 = Number To Fractional String(number=w3555, precision (6)=i16 2) -> (F-format string=w3556:string)  [unwired: 2 in]
                        n2522 = Concatenate Strings("Set Humidity [%RH] :" ("Content"), w3556) -> (w3558:string)
                        n2523 = local read "EVENT LOG"() -> (w3560:string)
                        n2524 = call "Event Log.vi"("Content"=w3558, "EVENT LOG"=w3560) -> ("EVENT LOG"=w3559:string)  [unwired: 8 in, 1 out]
                        n2525 = local write "EVENT LOG"(w3559) -> ()
                      }
                      frame #30 {
                        n2526 = Wait (ms)(milliseconds to wait=u32 50) -> ()  [unwired: 1 out]
                      }
                      frame #31 {
                        n2527 = local read "test time"() -> (w3563:dbl)
                        n2528 = Number To Fractional String(number=w3563, precision (6)=i16 1) -> (F-format string=w3564:string)  [unwired: 2 in]
                        n2529 = Concatenate Strings("Test Duration [mins] :" ("Content"), w3564) -> (w3566:string)
                        n2530 = local read "EVENT LOG"() -> (w3568:string)
                        n2531 = call "Event Log.vi"("Content"=w3566, "EVENT LOG"=w3568) -> ("EVENT LOG"=w3567:string)  [unwired: 8 in, 1 out]
                        n2532 = local write "EVENT LOG"(w3567) -> ()
                      }
                      frame #32 {
                        w3569 = dbl[] [] ("History Data")
                        w3570 = cluster{"y":dbl, dbl, "y":dbl}[] [] ("History Data")
                        w3571 = FALSE ("Visible")
                        n2533 = property on="Stroke ( mm )" class="WFChart (strict)"("History Data"=w3570) -> ()  [unwired: 2 in, 2 out]
                        n2534 = property on="Humidity ( %RH )" class="WFChart (strict)"("History Data"=w3569) -> ()  [unwired: 2 in, 2 out]
                        n2535 = property on="Temperature ( Deg C )" class="WFChart (strict)"("History Data"=w3569) -> ()  [unwired: 2 in, 2 out]
                        n2536 = property on="Electrical Contact Resistance ( % )" class="WFChart (strict)"("History Data"=w3569) -> ()  [unwired: 2 in, 2 out]
                        n2537 = property on="Coefficient of Friction" class="WFChart (strict)"("History Data"=w3569) -> ()  [unwired: 2 in, 2 out]
                        n2538 = property on="Frictional Force ( N )" class="WFChart (strict)"("History Data"=w3569) -> ()  [unwired: 2 in, 2 out]
                        n2539 = property on="Coefficient of Friction" class="WFChart (strict)"("History Data"=w3569) -> ()  [unwired: 2 in, 2 out]
                        n2540 = property on="Frictional Force ( N )" class="WFChart (strict)"("History Data"=w3569) -> ()  [unwired: 2 in, 2 out]
                        n2541 = property on="Electrical Contact Resistance ( % )" class="WFChart (strict)"("History Data"=w3569) -> ()  [unwired: 2 in, 2 out]
                        n2542 = property on="Humidity ( %RH )" class="WFChart (strict)"("History Data"=w3569) -> ()  [unwired: 2 in, 2 out]
                        n2543 = property on="Stroke ( mm )" class="WFChart (strict)"("History Data"=w3570) -> ()  [unwired: 2 in, 2 out]
                        n2544 = property on="Temperature ( Deg C )" class="WFChart (strict)"("History Data"=w3569) -> ()  [unwired: 2 in, 2 out]
                        n2545 = property on="Service Password Log" class="Str"("Visible"=w3571) -> ()  [unwired: 2 in, 2 out]
                        n2546 = property on="Password 3" class="Clust (strict)"("Visible"=w3571) -> ()  [unwired: 2 in, 2 out]
                      }
                    }
                    "TEST FILE NAM,E SAVED" <- TRUE ("TEST FILE NAM,E SAVED")
                  }
                }
              }
            }
          }
        }
        n2547 = case shown="True" w2868 {
          frame False {
            n2548 = local write "tfalg"(0.0 ("tfalg")) -> ()
          }
          frame True {
            n2549 = local read "tfalg"() -> (w3013:dbl)
            n2550 = Equal?(x=w3013, y=0.0) -> (x = y?=w3014:bool)
            n2551 = case shown="True" w3014 {
              frame False {
              }
              frame True {
                n2552 = local read "Total No. of Tests"() -> (w3017:dbl)
                n2553 = local write "tfalg"(1.0 ("tfalg")) -> ()
                n2554 = local write "acq 2"(FALSE ("acq 2")) -> ()
                n2555 = Wait (ms)(milliseconds to wait=u32 200) -> ()  [unwired: 1 out]
                n2556 = Increment(x=w3017) -> (x+1=w3016:dbl)
                n2557 = local write "Total No. of Tests"(w3016) -> ()
              }
            }
          }
        }
        n2558 = local write "Test \nStatus"(w2874) -> ()
        n2559 = local write "Save"(w2874) -> ()
        n2560 = local read "Main Tab"() -> (w2831:T2)
        n2561 = case shown="True" w2855 {
          tunnel: [FALSE ("RUN") TRUE ("RUN")] -> w2854
          tunnel: [_ 1] -> w2847
          frame False {
          }
          frame True {
          }
        }
        n2562 = In Range and Coerce(upper limit=w2862, x=w2835, lower limit=w2861) -> (In Range?=w2853:bool)  [unwired: 1 out]
        n2563 = In Range and Coerce(upper limit=w2859, x=w2834, lower limit=w2860) -> (In Range?=w2851:bool)  [unwired: 1 out]
        n2564 = case shown="True" w2867 {
          frame False {
            n2565 = local read "Rt 3"() -> (w2995:bool)
            n2566 = case shown="True" w2995 {
